vi "Requests.vi"(8 "error in (no error)":errorcluster, 9 "write enable":bool=TRUE, 11 "SMSD in":refnum<class "SMSD-DI.lvclass">) -> (0 "error out":errorcluster, 3 "SMSD out":refnum<class "SMSD-DI.lvclass">)   [LabVIEW 2021, in "SMSD-DI.lvclass"]
uses:
  SMSD-DI.lvclass
  D:/my_projects/projects/21/Master CR/Master CR.lvclass
  D:/my_projects/projects/21/Master CR/Devices/SMSD/SMSD.lvclass
  Master CR.lvclass/Master CR.ctl
  Data Unit/SMSD Data Unit/ERROR_OR_COMMANT_Type.ctl
  Data Unit/SMSD Data Unit/SMSD Data Unit.lvclass/SMSD Data Unit.ctl
  Network Protocol/SMSD Master/SMSD Master.lvclass/SMSD Master.ctl
  Transmission Data Unit/SMSD/SMSD ADU.lvclass/SMSD ADU.ctl
  SMSD_cmd_Data_format.vi
  Data Unit/SMSD Data Unit/Construct PDU.vi
  Network Protocol/SMSD Master/Read write Master.vi
  Data Unit/SMSD Data Unit/Deconstruct PDU.vi
  Network Protocol/Read Network Protocol.vi
  Transmission Data Unit/SMSD/Write ADU Packet.vi
  Transmission Data Unit/SMSD/Read ADU Packet.vi
  Modbus_v121c/Network Interface/TCP Interface/TSC/TCP Write.vi
  Data Unit/SMSD Data Unit/Flatten PDU.vi
  Data Unit/SMSD Data Unit/Unflatten to PDU.vi
  Modbus_v121c/Network Interface/TCP Interface/TSC/TCP Read.vi
  <vilib>/Utility/error.llb/Clear Errors.vi
  SMSD.lvclass
  Network Protocol/SMSD Master/SMSD Master.lvclass
  Data Unit/SMSD Data Unit/SMSD Data Unit.lvclass
  Modbus_v121c/Data Model/Device Data Model.lvclass
  Master CR.lvclass
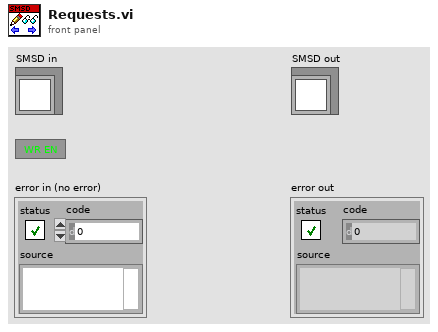
[diagram p1: front panel]
types:
  T1 = enum8{"CMD_PowerSTEP01_END", "CMD_PowerSTEP01_GET_SPEED", "CMD_PowerSTEP01_STATUS_IN_EVENT", "CMD_PowerSTEP01_SET_MODE", "CMD_PowerSTEP01_GET_MODE", "CMD_PowerSTEP01_SET_MIN_SPEED", "CMD_PowerSTEP01_SET_MAX_SPEED", "CMD_PowerSTEP01_SET_ACC", "CMD_PowerSTEP01_SET_DEC", "CMD_PowerSTEP01_SET_FS_SPEED", "CMD_PowerSTEP01_SET_MASK_EVENT", "CMD_PowerSTEP01_GET_ABS_POS", "CMD_PowerSTEP01_GET_EL_POS", "CMD_PowerSTEP01_GET_STATUS_AND_CLR", "CMD_PowerSTEP01_RUN_F", "CMD_PowerSTEP01_RUN_R", "CMD_PowerSTEP01_MOVE_F", "CMD_PowerSTEP01_MOVE_R", "CMD_PowerSTEP01_GO_TO_F", "CMD_PowerSTEP01_GO_TO_R", "CMD_PowerSTEP01_GO_UNTIL_F", "CMD_PowerSTEP01_GO_UNTIL_R", "CMD_PowerSTEP01_SCAN_ZERO_F", "CMD_PowerSTEP01_SCAN_ZERO_R", "CMD_PowerSTEP01_SCAN_LABEL_F", "CMD_PowerSTEP01_SCAN_LABEL_R", "CMD_PowerSTEP01_GO_ZERO", "CMD_PowerSTEP01_GO_LABEL", "CMD_PowerSTEP01_GO_TO", "CMD_PowerSTEP01_RESET_POS", "CMD_PowerSTEP01_RESET_POWERSTEP01", "CMD_PowerSTEP01_SOFT_STOP", "CMD_PowerSTEP01_HARD_STOP", "CMD_PowerSTEP01_SOFT_HI_Z", "CMD_PowerSTEP01_HARD_HI_Z", "CMD_PowerSTEP01_SET_WAIT", "CMD_PowerSTEP01_SET_RELE", "CMD_PowerSTEP01_CLR_RELE", "CMD_PowerSTEP01_GET_RELE", "CMD_PowerSTEP01_WAIT_IN0", "CMD_PowerSTEP01_WAIT_IN1", "CMD_PowerSTEP01_GOTO_PROGRAM", "CMD_PowerSTEP01_GOTO_PROGRAM_IF_IN0", "CMD_PowerSTEP01_GOTO_PROGRAM_IF_IN1", "CMD_PowerSTEP01_LOOP_PROGRAM", "CMD_PowerSTEP01_CALL_PROGRAM", "CMD_PowerSTEP01_RETURN_PROGRAM", "CMD_PowerSTEP01_START_PROGRAM_MEM0", "CMD_PowerSTEP01_START_PROGRAM_MEM1", "CMD_PowerSTEP01_START_PROGRAM_MEM2", "CMD_PowerSTEP01_START_PROGRAM_MEM3", "CMD_PowerSTEP01_STOP_PROGRAM_MEM", "CMD_PowerSTEP01_STEP_CLOCK", "CMD_PowerSTEP01_STOP_USB", "CMD_PowerSTEP01_GET_MIN_SPEED", "CMD_PowerSTEP01_GET_MAX_SPEED", "CMD_PowerSTEP01_GET_STACK", "CMD_PowerSTEP01_GOTO_PROGRAM_IF_ZERO", "CMD_PowerSTEP01_GOTO_PROGRAM_IF_IN_ZERO", "CMD_PowerSTEP01_WAIT_CONTINUE", "CMD_PowerSTEP01_SET_WAIT_2", "CMD_PowerSTEP01_SCAN_MARK2_F", "CMD_PowerSTEP01_SCAN_MARK2_R"}
  T2 = typedef "SMSD Data Unit.lvclass/ERROR_OR_COMMANT_Type.ctl" = enum8{"OK", "OK_ACCESS", "ERROR_ACCESS", "ERROR_ACCESS_TIMEOUT", "ERROR_XOR", "ERROR_NO_COMMAND", "ERROR_LEN", "ERROR_RANGE", "ERROR_WRITE", "ERROR_READ", "ERROR_PROGRAMS", "ERROR_WRITE_SETUP", "NO_NEXT", "END_PROGRAMS", "COMMAND_GET_STATUS_IN_EVENT", "COMMAND_GET_MODE", "COMMAND_GET_ABS_POS", "COMMAND_GET_EL_POS", "COMMAND_GET_SPEED", "COMMAND_GET_MIN_SPEED", "COMMAND_GET_MAX_SPEED", "COMMAND_GET_STACK", "STATUS_RELE_SET", "STATUS_RELE_CLR"}
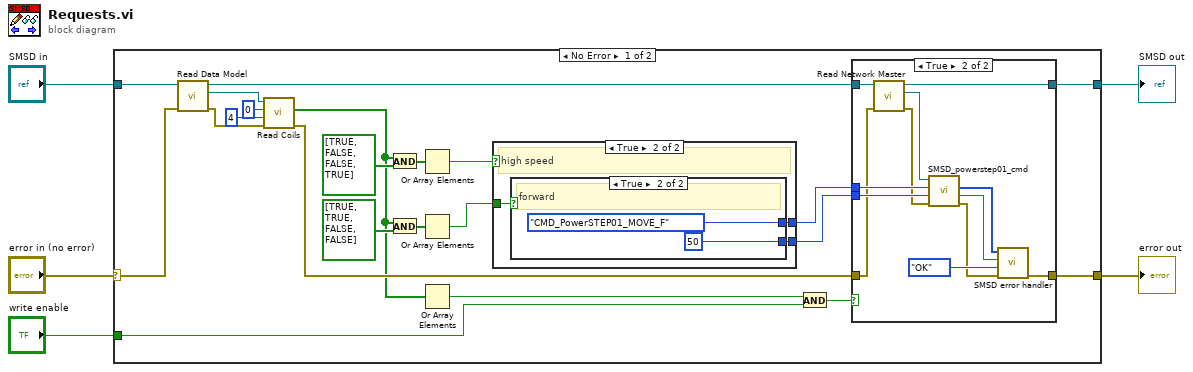
[diagram p0: block diagram]
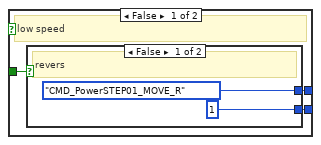
[diagram p2: hidden frame]
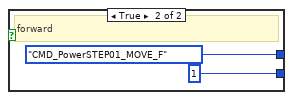
[diagram p3: hidden frame]
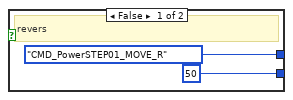
[diagram p4: hidden frame]
diagram:
  n1 = case shown="No Error" "error in (no error)" {
    selector: "error in (no error)" -> [w13 w57]
    tunnel: [w26 w57] -> w1
    tunnel: [w27 w56] -> w2
    tunnel: "SMSD in" -> [w14 w56]
    tunnel: "write enable" -> [w16 _]
    frame No Error {
      n2 = call "Read Data Model.vi"("error in (no error)"=w13, "Master CR in"=w14) -> ("error out"=w11:errorcluster, "Data Model"=w9:refnum<class "Device Data Model.lvclass">, "Master CR out"=w12:refnum<class "SMSD-DI.lvclass">)  [unwired: 7 in]
      n3 = call-dynamic "Read Coils.vi"("error in"=w11, "number of coils"=u16 4, "starting address"=u16 0, "device data model in"=w9) -> ("error out"=w10:errorcluster, "data"=w6:bool[])  [unwired: 5 in, 1 out]
      n4 = And(x=w6, y=bool[] [TRUE, FALSE, FALSE, TRUE] ("x")) -> (x .and. y?=w25:bool[])
      n5 = And(x=w6, y=bool[] [TRUE, TRUE, FALSE, FALSE] ("x")) -> (x .and. y?=w22:bool[])
      n6 = Or Array Elements(Boolean array=w25) -> (logical OR=w21:bool)
      n7 = Or Array Elements(Boolean array=w22) -> (logical OR=w20:bool)
      n8 = Or Array Elements(Boolean array=w6) -> (logical OR=w15:bool)
      n9 = case shown="True" w21 {
        tunnel: w20 -> [w30 w37]
        tunnel: [w29 w36] -> w19
        tunnel: [w28 w35] -> w18
        frame False {
          # "low speed"
          n10 = case shown="False" w30 {
            tunnel: [T1."CMD_PowerSTEP01_MOVE_R" ("COMMAND (END)") T1."CMD_PowerSTEP01_MOVE_F" ("COMMAND (END)")] -> w29
            tunnel: [u32 1 ("DATA (0)") u32 1 ("DATA (0)")] -> w28
            frame False {
              # "revers"
            }
            frame True {
              # "forward"
            }
          }
        }
        frame True {
          # "high speed"
          n11 = case shown="True" w37 {
            tunnel: [T1."CMD_PowerSTEP01_MOVE_R" ("COMMAND (END)") T1."CMD_PowerSTEP01_MOVE_F" ("COMMAND (END)")] -> w36
            tunnel: [u32 50 ("DATA (0)") u32 50 ("DATA (0)")] -> w35
            frame False {
              # "revers"
            }
            frame True {
              # "forward"
            }
          }
        }
      }
      n12 = And(x=w15, y=w16) -> (x .and. y?=w17:bool)
      n13 = case shown="True" w17 {
        tunnel: [w43 w44] -> w27
        tunnel: w12 -> [w43 w48]
        tunnel: [w42 w51] -> w26
        tunnel: w10 -> [w42 w46]
        tunnel: w19 -> [_ w50]
        tunnel: w18 -> [_ w49]
        frame False {
        }
        frame True {
          n14 = call "Read Network Master.vi"("error in (no error)"=w46, "SMSD in"=w48) -> ("error out"=w45:errorcluster, "TCP Master"=w47:refnum<class "SMSD Master.lvclass">, "SMSD out"=w44:refnum<class "SMSD-DI.lvclass">)  [unwired: 7 in]
          n15 = call "SMSD_powerstep01_cmd.vi"("error in (no error)"=w45, "DATA (0)"=w49, "COMMAND (END)"=w50, "SMSD in"=w47) -> ("error out"=w52:errorcluster, "PDU valid?"=w53:bool, "data"=w55:u8[])  [unwired: 4 in, 1 out]
          n16 = call "SMSD error handler.vi"("error in (no error)"=w52, "correct answer (OK)"=ERROR_OR_COMMANT_Type."OK" ("coerced x 2"), "timed out?"=w53, "data"=w55) -> ("error out"=w51:errorcluster)  [unwired: 7 in]
        }
      }
    }
    frame Error {
    }
  }
  "error out" <- w1
  "SMSD out" <- w2
